vi "Read Sleep Limits (ns).vi"(8 "error in (no error)":errorcluster, 11 "CIFCorePlugin in":refnum<class "CIFCorePlugin.lvclass">) -> (0 "error out":errorcluster, 2 "FTE Limits (ns)":T1={"Maximum"=200000000, "Minimum"=20000} {"Maximum" format="%.0e"; "Minimum" format="%.0e"}, 3 "CIFCorePlugin out":refnum<class "CIFCorePlugin.lvclass">)   [LabVIEW 2021, in "CIFCorePlugin.lvclass"]
uses:
  CIFCorePlugin.lvclass
  CIFUtilities/CIFClocks/Typedef/Future Time Event Limits.ctl
  CIFCorePlugin.lvclass/CIFCorePlugin.ctl
  CIFUtilities/CIFClocks/CIFClocks.lvlib
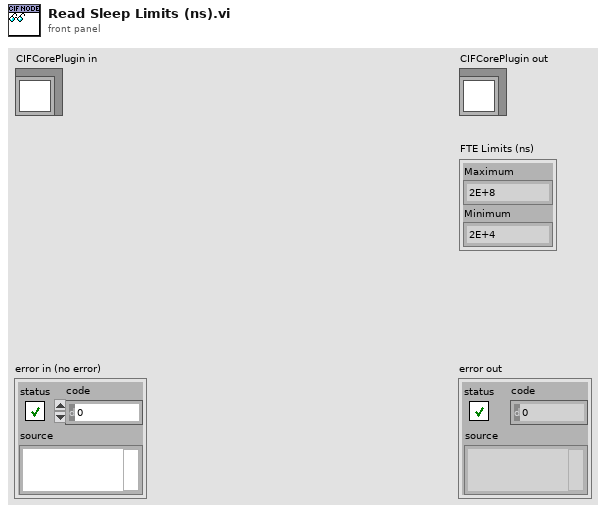
[diagram p1: front panel]
types:
  T1 = typedef "CIFClocks.lvlib/Future Time Event Limits.ctl" = cluster{"Maximum":u64, "Minimum":u64}
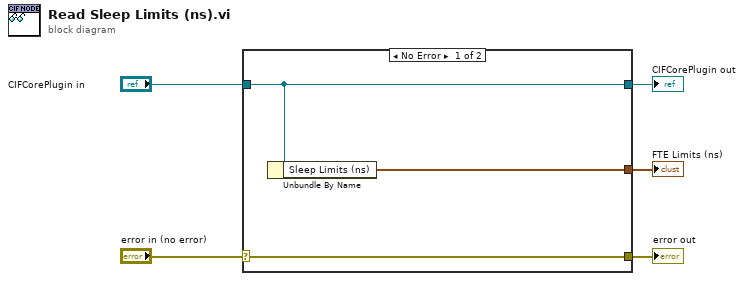
[diagram p0: block diagram]
diagram:
  n1 = case shown="No Error" "error in (no error)" {
    selector: "error in (no error)" -> [w8 w9]
    tunnel: [w8 w9] -> w4
    tunnel: [w7 w10] -> w2
    tunnel: "CIFCorePlugin in" -> [w7 w10]
    tunnel: [w6 _] -> w1
    frame No Error {
      n2 = Unbundle By Name(w7) -> ("Sleep Limits (ns)"=w6:T1)
    }
    frame Error {
    }
  }
  "error out" <- w4
  "CIFCorePlugin out" <- w2
  "FTE Limits (ns)" <- w1
